vi "AB_820_850_Project_Source_ExportedVI.vi"(6 "dataForPrevious":T2, 7 "action":T6, 8 "error in (no error)":errorcluster, 9 "index in":i32, 10 "dataSource in":cluster{"vipInfo":T1}, 11 "buildObject":T5) -> (0 "error out":errorcluster, 1 "index out":i32, 2 "dataSource out":cluster{"vipInfo":T1}, 3 "buildObject out":T5)   [LabVIEW 2020]
doc: "Reads and writes the data to the object property bag."
uses:
  <resource>/Framework/Providers/API/ItemRef.ctl
  <vilib>/AppBuilder/RW_Project/AB_RW_Project_PropBag_Action.ctl
  <vilib>/AppBuilder/RW_Project/AB_RW_Project_Source_Data_for_Previous.ctl
  <vilib>/AppBuilder/AB_BuildType.ctl
  <vilib>/Utility/lvfile.llb/LVFileType.ctl
  <vilib>/AppBuilder/ABAPI Dist VI Proto Info.ctl
  <vilib>/Utility/lvfile.llb/NI_FileType.lvlib
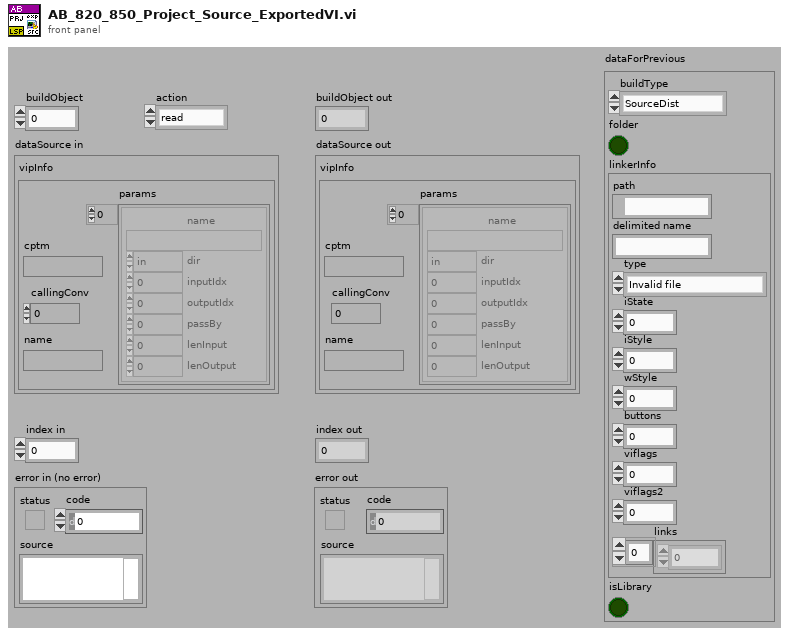
[diagram p1: front panel]
types:
  T1 = typedef "ABAPI Dist VI Proto Info.ctl" = cluster{"cptm":string, "params":cluster{"name":string, "dir":enum32{"in", "out", "in/out", "length"}, "inputIdx":i32, "outputIdx":i32, "passBy":i32, "lenInput":i32, "lenOutput":i32}[], "callingConv":i32, "name":string}
  T2 = typedef "AB_RW_Project_Source_Data_for_Previous.ctl" = cluster{"buildType":T3, "folder":bool, "linkerInfo":cluster{"path":path, "delimited name":string, "type":T4, "iState":u32, "iStyle":u16, "wStyle":u16, "buttons":u16, "viflags":u32, "viflags2":u32, "links":u32[]}, "isLibrary":bool}
  T3 = typedef "AB_BuildType.ctl" = enum16{"SourceDist", "EXE", "DLL", "RTExe"}
  T4 = typedef "NI_FileType.lvlib/LVFileType.ctl" = enum32{"Invalid file", "Unknown type", "Instrument", "Control", "Polymorphic VI", "Project", "Library", "LVClass", "XControl", "XNode", "Shared library", ".NET assembly", "ActiveX interface", "CIN", "Run-time menu", "Palette menu", "Help file", "LLB", "XNode Edit Dependency", "Class Private Data Control", "Statechart", "MathScript .m file", "Ladder Diagram", "LVLibp", "XNode Build Dependency"}
  T5 = typedef "ItemRef.ctl" = u64
  T6 = typedef "AB_RW_Project_PropBag_Action.ctl" = enum16{"read", "write", "clear", "readPrevious", "writePrevious", "clearPrevious"}
  T7 = cluster{"name":string, "dir":enum32{"in", "out", "in/out", "length"}, "inputIdx":i32, "outputIdx":i32, "passBy":i32, "lenInput":i32, "lenOutput":i32}
  T8 = cluster{"name":string, "dir":enum32{"in", "out", "in/out", "length"}, "inputIdx":i32, "outputIdx":i32, "passBy":i32, "lenInput":i32, "lenOutput":i32}[]
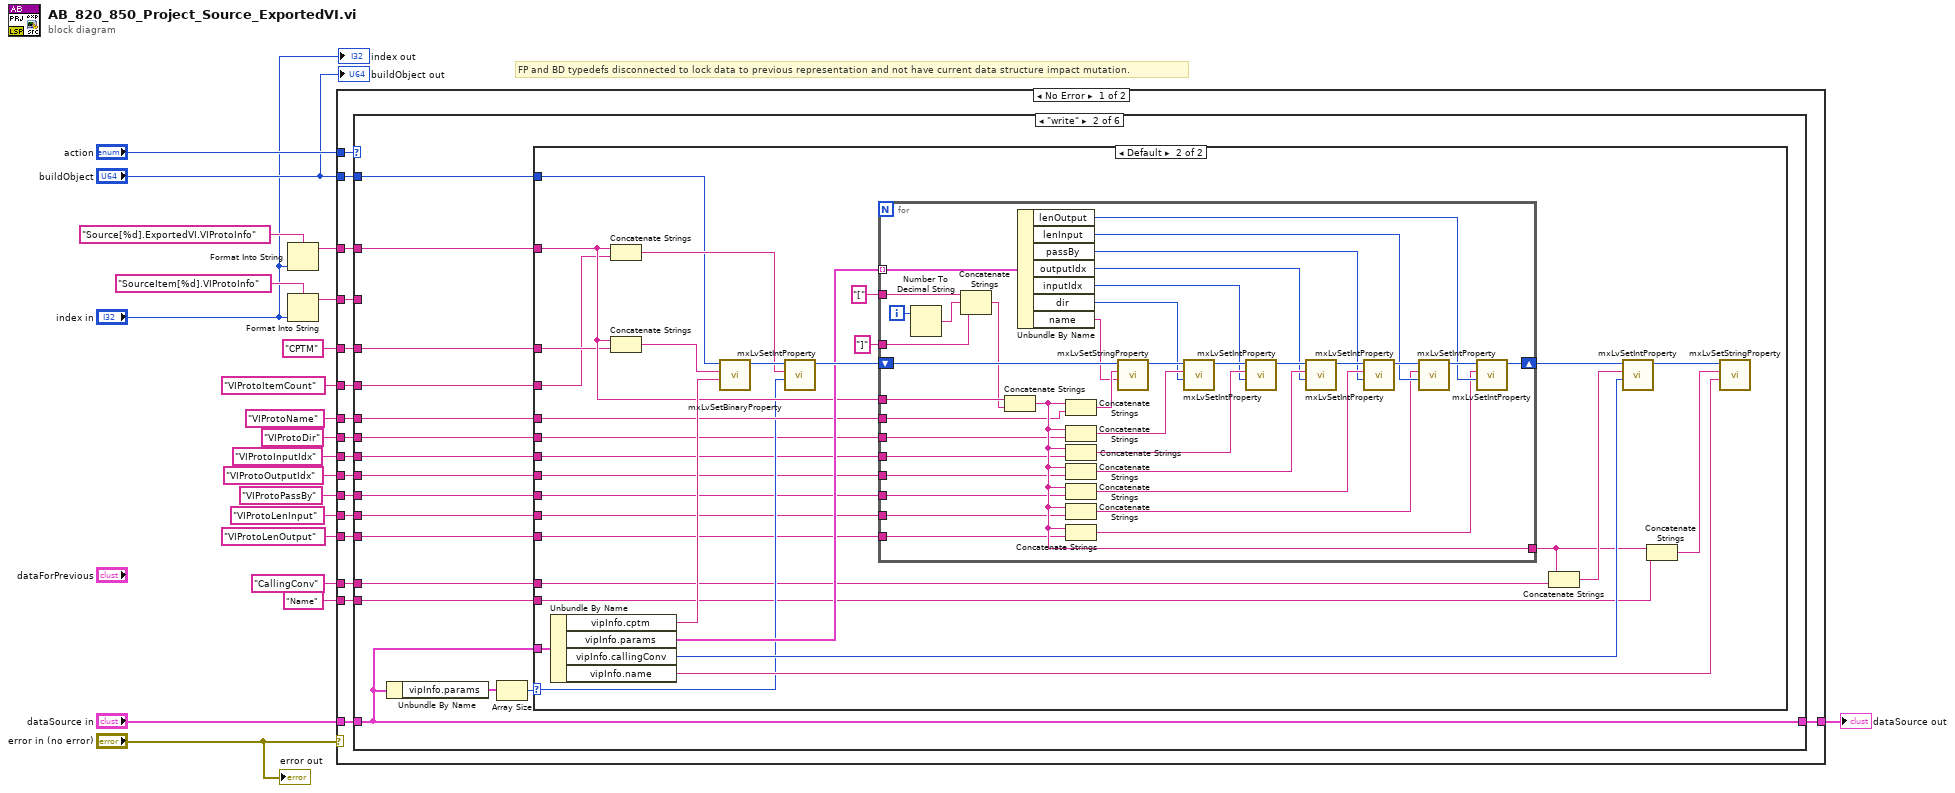
[diagram p0: block diagram]
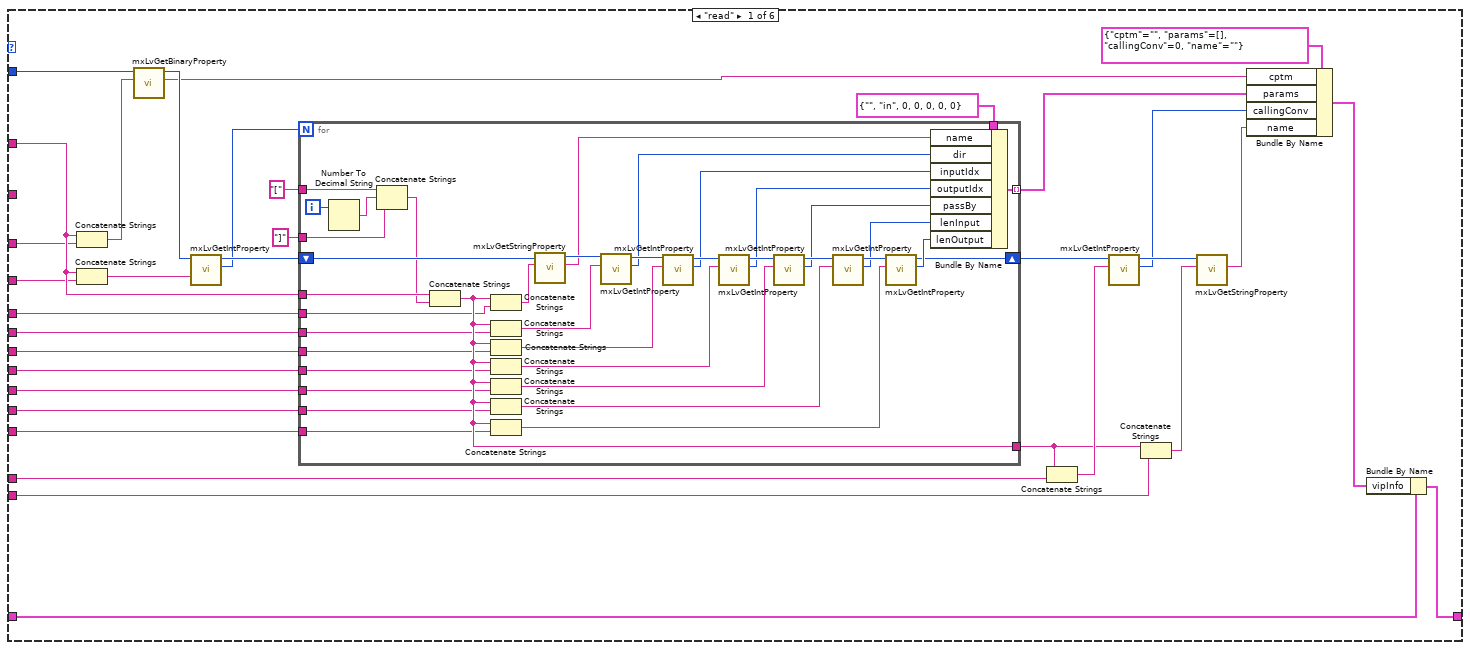
[diagram p2: hidden frame]
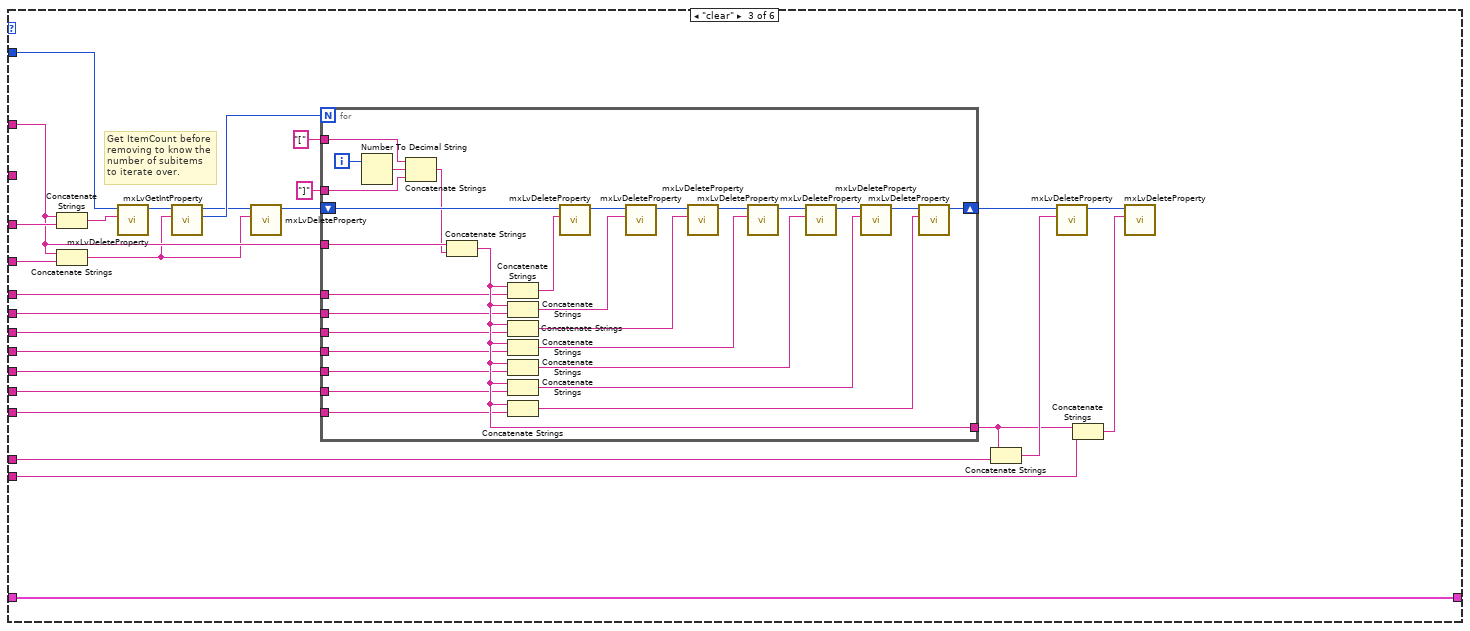
[diagram p4: hidden frame]
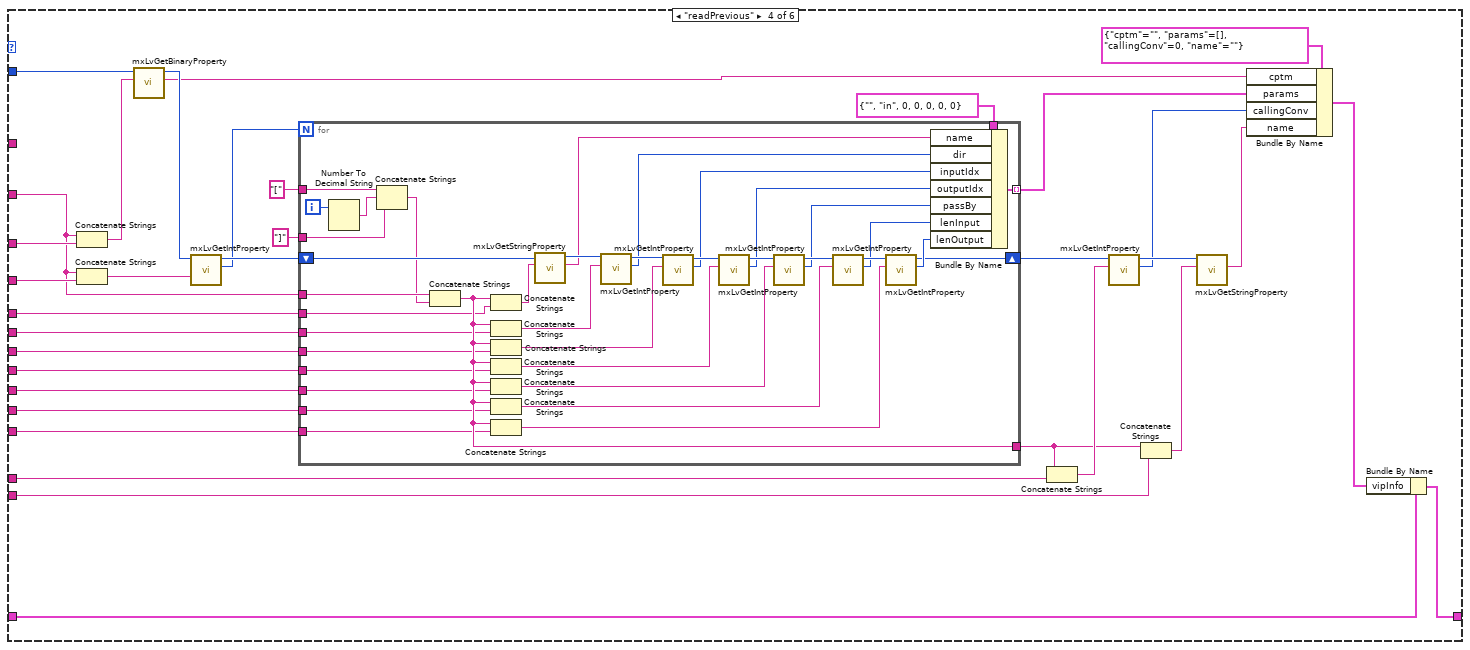
[diagram p5: hidden frame]
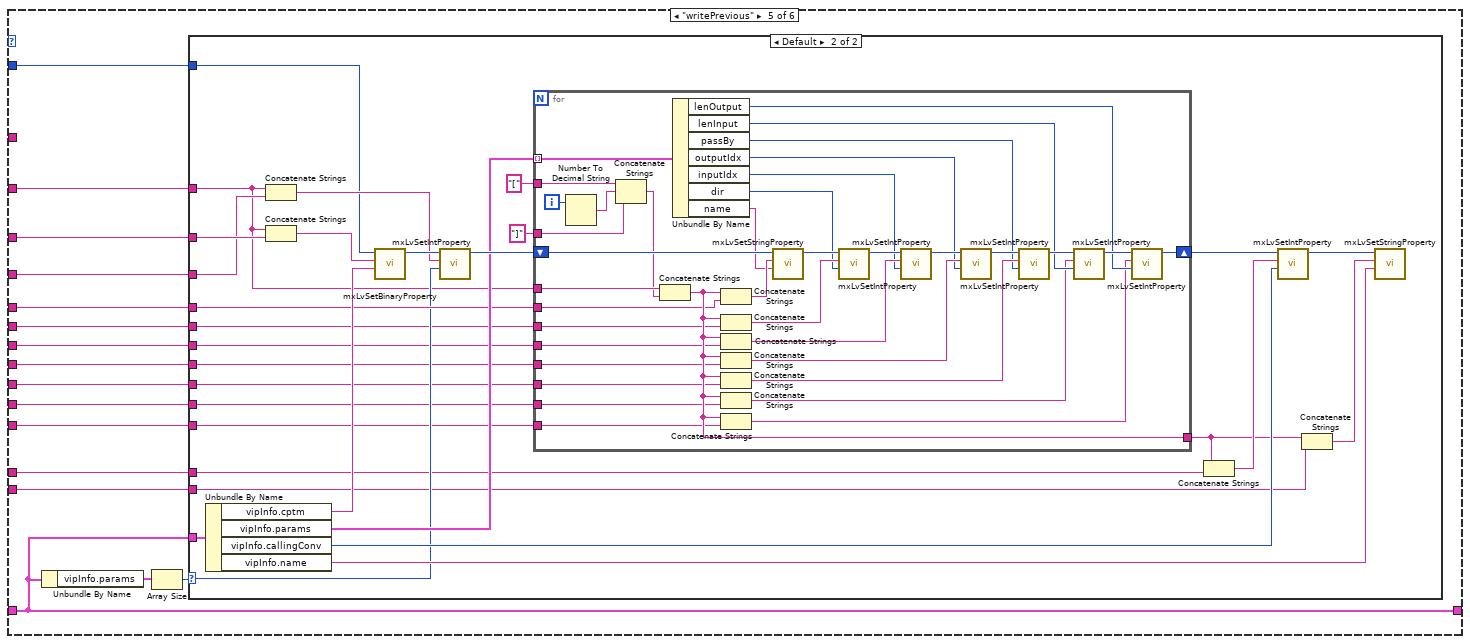
[diagram p6: hidden frame]
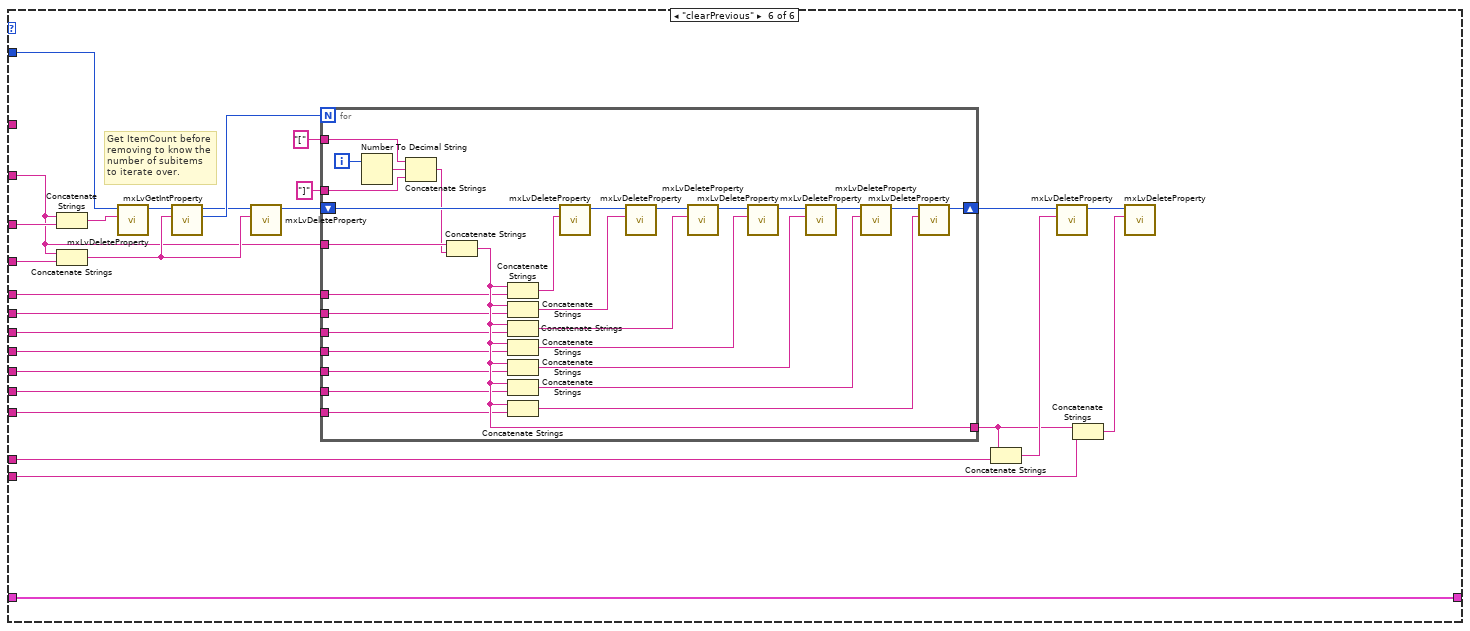
[diagram p8: hidden frame]
diagram:
  # "FP and BD typedefs disconnected to lock data to previous representation and not have current data structure impact mutation."
  n1 = Format Into String(format string="Source[%d].ExportedVI.VIProtoInfo", "index in") -> (resulting string=w19:string)  [unwired: 2 in, 1 out]
  n2 = Format Into String(format string="SourceItem[%d].VIProtoInfo", "index in") -> (resulting string=w17:string)  [unwired: 2 in, 1 out]
  n3 = case shown="No Error" "error in (no error)" {
    tunnel: "action" -> [w38 _]
    tunnel: "dataSource in" -> [w37 w461]
    tunnel: w19 -> [w36 _]
    tunnel: w17 -> [w35 _]
    tunnel: "buildObject" -> [w34 _]
    tunnel: [w33 w461] -> w12
    tunnel: "CPTM" -> [w32 _]
    tunnel: "VIProtoItemCount" -> [w31 _]
    tunnel: "VIProtoName" ("string") -> [w30 _]
    tunnel: "VIProtoDir" ("string") -> [w29 _]
    tunnel: "VIProtoInputIdx" ("string") -> [w28 _]
    tunnel: "VIProtoOutputIdx" ("string") -> [w27 _]
    tunnel: "VIProtoPassBy" ("string") -> [w26 _]
    tunnel: "VIProtoLenInput" ("string") -> [w25 _]
    tunnel: "VIProtoLenOutput" ("string") -> [w24 _]
    tunnel: "CallingConv" -> [w23 _]
    tunnel: "Name" -> [w22 _]
    frame No Error {
      n4 = case shown="\"write\"" w38 {
        tunnel: w34 -> [w69 w124 w217 w281 w336 w429]
        tunnel: w37 -> [w72 w119 w220 w283 w331 w431]
        tunnel: w36 -> [w70 w125 w218 _ _ _]
        tunnel: w35 -> [_ _ _ w250 w322 w405]
        tunnel: [w71 w119 w220 w282 w331 w431] -> w33
        tunnel: w32 -> [w49 w122 w219 w261 w334 w430]
        tunnel: w31 -> [w48 w121 w216 w260 w333 w428]
        tunnel: w30 -> [w47 w123 w202 w259 w335 w414]
        tunnel: w29 -> [w46 w118 w201 w258 w330 w413]
        tunnel: w28 -> [w45 w117 w200 w257 w329 w412]
        tunnel: w27 -> [w44 w116 w199 w256 w328 w411]
        tunnel: w26 -> [w43 w115 w198 w255 w327 w410]
        tunnel: w25 -> [w42 w114 w197 w254 w326 w409]
        tunnel: w24 -> [w41 w113 w196 w253 w325 w408]
        tunnel: w23 -> [w40 w112 w194 w252 w324 w406]
        tunnel: w22 -> [w39 w111 w195 w251 w323 w407]
        frame "read" {
          n5 = Concatenate Strings(w70, w49) -> (w66:string)
          n6 = Concatenate Strings(w70, w48) -> (w62:string)
          n7 = call <resource>:"mxLvGetBinaryProperty.vi"("Tag"=w66, "Item"=w69) -> ("Value"=w50:string, "Item"=w63:T5)  [unwired: 7 in, 1 out]
          n8 = call <resource>:"mxLvGetIntProperty.vi"("Tag"=w62, "Item"=w63) -> ("Value"=w56:i32, "Item"=w61:T5)  [unwired: 7 in, 1 out]
          n9 = for {
            N: w56 -> [_]
            tunnel: "[" -> [w109]
            tunnel: "]" -> [w108]
            tunnel: w70 -> [w103]
            tunnel: [w90] -> w57
            tunnel: T7 {"name"="", "dir"=enum."in", "inputIdx"=0, "outputIdx"=0, "passBy"=0, "lenInput"=0, "lenOutput"=0} -> [w89]
            tunnel: [w81] -> w53 mode=indexing
            shift-right: [w80] -> w51
            shift-left: w61 -> [w106]
            tunnel: w47 -> [w79]
            tunnel: w46 -> [w78]
            tunnel: w45 -> [w77]
            tunnel: w44 -> [w76]
            tunnel: w43 -> [w75]
            tunnel: w42 -> [w74]
            tunnel: w41 -> [w73]
            i -> [w107]
            n10 = Number To Decimal String(number=w107) -> (decimal integer string=w110:string)  [unwired: 1 in]
            n11 = Concatenate Strings(w109, w110, w108) -> (w102:string)
            n12 = Concatenate Strings(w103, w102) -> (w90:string)
            n13 = Concatenate Strings(w90, w79) -> (w105:string)
            n14 = Concatenate Strings(w90, w78) -> (w101:string)
            n15 = Concatenate Strings(w90, w77) -> (w100:string)
            n16 = Concatenate Strings(w90, w76) -> (w94:string)
            n17 = Concatenate Strings(w90, w75) -> (w93:string)
            n18 = Concatenate Strings(w90, w74) -> (w92:string)
            n19 = Concatenate Strings(w90, w73) -> (w91:string)
            n20 = call <resource>:"mxLvGetStringProperty.vi"("Tag"=w105, "Item"=w106) -> ("Value"=w88:string, "Item"=w104:T5)  [unwired: 7 in, 1 out]
            n21 = call <resource>:"mxLvGetIntProperty.vi"("Tag"=w101, "Item"=w104) -> ("Value"=w87:i32, "Item"=w99:T5)  [unwired: 7 in, 1 out]
            n22 = call <resource>:"mxLvGetIntProperty.vi"("Tag"=w100, "Item"=w99) -> ("Value"=w86:i32, "Item"=w98:T5)  [unwired: 7 in, 1 out]
            n23 = call <resource>:"mxLvGetIntProperty.vi"("Tag"=w94, "Item"=w98) -> ("Value"=w85:i32, "Item"=w97:T5)  [unwired: 7 in, 1 out]
            n24 = call <resource>:"mxLvGetIntProperty.vi"("Tag"=w93, "Item"=w97) -> ("Value"=w84:i32, "Item"=w96:T5)  [unwired: 7 in, 1 out]
            n25 = call <resource>:"mxLvGetIntProperty.vi"("Tag"=w92, "Item"=w96) -> ("Value"=w83:i32, "Item"=w95:T5)  [unwired: 7 in, 1 out]
            n26 = call <resource>:"mxLvGetIntProperty.vi"("Tag"=w91, "Item"=w95) -> ("Value"=w82:i32, "Item"=w80:T5)  [unwired: 7 in, 1 out]
            n27 = Bundle By Name(cluster=w89, "name"=w88, "dir"=w87, "inputIdx"=w86, "outputIdx"=w85, "passBy"=w84, "lenInput"=w83, "lenOutput"=w82) -> (w81:T7)
          }
          n28 = Concatenate Strings(w57, w40) -> (w64:string)
          n29 = call <resource>:"mxLvGetIntProperty.vi"("Tag"=w64, "Item"=w51) -> ("Value"=w54:i32, "Item"=w58:T5)  [unwired: 7 in, 1 out]
          n30 = Concatenate Strings(w57, w39) -> (w65:string)
          n31 = call <resource>:"mxLvGetStringProperty.vi"("Tag"=w65, "Item"=w58) -> ("Value"=w52:string)  [unwired: 7 in, 2 out]
          n32 = Bundle By Name(cluster=T1 {"cptm"="", "params"=[], "callingConv"=0, "name"=""} ("vipInfo"), "cptm"=w50, "params"=w53, "callingConv"=w54, "name"=w52) -> (w67:T1)
          n33 = Bundle By Name(cluster=w72, "vipInfo"=w67) -> (w71:cluster{"vipInfo":T1})
        }
        frame "write" {
          n34 = Unbundle By Name(w119) -> ("vipInfo.params"=w126:T8)
          n35 = Array Size(array=w126) -> (size(s)=w120:i32)
          n36 = case shown="Default" w120 {
            selector: w120 -> [_ w135]
            tunnel: w124 -> [_ w141]
            tunnel: w119 -> [_ w140]
            tunnel: w125 -> [_ w139]
            tunnel: w123 -> [_ w138]
            tunnel: w122 -> [_ w137]
            tunnel: w121 -> [_ w136]
            tunnel: w118 -> [_ w134]
            tunnel: w117 -> [_ w133]
            tunnel: w116 -> [_ w132]
            tunnel: w115 -> [_ w131]
            tunnel: w114 -> [_ w130]
            tunnel: w113 -> [_ w129]
            tunnel: w112 -> [_ w128]
            tunnel: w111 -> [_ w127]
            frame 0 {
              # "If default, then don't write anything out."
            }
            frame Default {
              n37 = Unbundle By Name(w140) -> ("vipInfo.cptm"=w155:string, "vipInfo.params"=w147:T8, "vipInfo.callingConv"=w151:i32, "vipInfo.name"=w152:string)
              n38 = Concatenate Strings(w139, w136) -> (w149:string)
              n39 = Concatenate Strings(w139, w137) -> (w156:string)
              n40 = call <resource>:"mxLvSetBinaryProperty.vi"("Value"=w155, "Tag"=w156, "Item"=w141) -> ("Item"=w150:T5)  [unwired: 7 in, 1 out]
              n41 = call <resource>:"mxLvSetIntProperty.vi"("Value (0)"=w135, "Tag"=w149, "Item"=w150) -> ("Item"=w148:T5)  [unwired: 7 in, 1 out]
              n42 = for {
                tunnel: w147 -> [w193] mode=indexing
                tunnel: "[" -> [w191]
                tunnel: "]" -> [w190]
                tunnel: w139 -> [w184]
                tunnel: [w165] -> w142
                shift-right: [w164] -> w144
                shift-left: w148 -> [w188]
                tunnel: w138 -> [w163]
                tunnel: w134 -> [w162]
                tunnel: w133 -> [w161]
                tunnel: w132 -> [w160]
                tunnel: w131 -> [w159]
                tunnel: w130 -> [w158]
                tunnel: w129 -> [w157]
                i -> [w189]
                n43 = Number To Decimal String(number=w189) -> (decimal integer string=w192:string)  [unwired: 1 in]
                n44 = Concatenate Strings(w191, w192, w190) -> (w183:string)
                n45 = Concatenate Strings(w184, w183) -> (w165:string)
                n46 = Unbundle By Name(w193) -> ("lenOutput"=w167:i32, "lenInput"=w169:i32, "passBy"=w170:i32, "outputIdx"=w171:i32, "inputIdx"=w178:i32, "dir"=w181:enum32{"in", "out", "in/out", "length"}, "name"=w186:string)
                n47 = Concatenate Strings(w165, w163) -> (w187:string)
                n48 = Concatenate Strings(w165, w162) -> (w182:string)
                n49 = Concatenate Strings(w165, w161) -> (w180:string)
                n50 = Concatenate Strings(w165, w160) -> (w173:string)
                n51 = Concatenate Strings(w165, w159) -> (w172:string)
                n52 = Concatenate Strings(w165, w158) -> (w168:string)
                n53 = Concatenate Strings(w165, w157) -> (w166:string)
                n54 = call <resource>:"mxLvSetStringProperty.vi"("Value (\"\")"=w186, "Tag"=w187, "Item"=w188) -> ("Item"=w185:T5)  [unwired: 7 in, 1 out]
                n55 = call <resource>:"mxLvSetIntProperty.vi"("Value (0)"=w181, "Tag"=w182, "Item"=w185) -> ("Item"=w179:T5)  [unwired: 7 in, 1 out]
                n56 = call <resource>:"mxLvSetIntProperty.vi"("Value (0)"=w178, "Tag"=w180, "Item"=w179) -> ("Item"=w177:T5)  [unwired: 7 in, 1 out]
                n57 = call <resource>:"mxLvSetIntProperty.vi"("Value (0)"=w171, "Tag"=w173, "Item"=w177) -> ("Item"=w176:T5)  [unwired: 7 in, 1 out]
                n58 = call <resource>:"mxLvSetIntProperty.vi"("Value (0)"=w170, "Tag"=w172, "Item"=w176) -> ("Item"=w175:T5)  [unwired: 7 in, 1 out]
                n59 = call <resource>:"mxLvSetIntProperty.vi"("Value (0)"=w169, "Tag"=w168, "Item"=w175) -> ("Item"=w174:T5)  [unwired: 7 in, 1 out]
                n60 = call <resource>:"mxLvSetIntProperty.vi"("Value (0)"=w167, "Tag"=w166, "Item"=w174) -> ("Item"=w164:T5)  [unwired: 7 in, 1 out]
              }
              n61 = Concatenate Strings(w142, w128) -> (w153:string)
              n62 = call <resource>:"mxLvSetIntProperty.vi"("Value (0)"=w151, "Tag"=w153, "Item"=w144) -> ("Item"=w143:T5)  [unwired: 7 in, 1 out]
              n63 = Concatenate Strings(w142, w127) -> (w154:string)
              n64 = call <resource>:"mxLvSetStringProperty.vi"("Value (\"\")"=w152, "Tag"=w154, "Item"=w143) -> ()  [unwired: 7 in, 2 out]
            }
          }
        }
        frame "clear" {
          # "Get ItemCount before removing to know the number of subitems to iterate over."
          n65 = Concatenate Strings(w218, w219) -> (w215:string)
          n66 = Concatenate Strings(w218, w216) -> (w203:string)
          n67 = call <resource>:"mxLvDeleteProperty.vi"("Tag"=w215, "Item"=w217) -> ("Item"=w205:T5)  [unwired: 8 in, 1 out]
          n68 = call <resource>:"mxLvGetIntProperty.vi"("Tag"=w203, "Item"=w205) -> ("Value"=w206:i32, "Item"=w204:T5)  [unwired: 7 in, 1 out]
          n69 = call <resource>:"mxLvDeleteProperty.vi"("Tag"=w203, "Item"=w204) -> ("Item"=w212:T5)  [unwired: 8 in, 1 out]
          n70 = for {
            N: w206 -> [_]
            tunnel: "[" -> [w248]
            tunnel: "]" -> [w247]
            tunnel: w218 -> [w242]
            tunnel: [w229] -> w207
            shift-right: [w228] -> w209
            shift-left: w212 -> [w245]
            tunnel: w202 -> [w227]
            tunnel: w201 -> [w226]
            tunnel: w200 -> [w225]
            tunnel: w199 -> [w224]
            tunnel: w198 -> [w223]
            tunnel: w197 -> [w222]
            tunnel: w196 -> [w221]
            i -> [w246]
            n71 = Number To Decimal String(number=w246) -> (decimal integer string=w249:string)  [unwired: 1 in]
            n72 = Concatenate Strings(w248, w249, w247) -> (w241:string)
            n73 = Concatenate Strings(w242, w241) -> (w229:string)
            n74 = Concatenate Strings(w229, w227) -> (w244:string)
            n75 = Concatenate Strings(w229, w226) -> (w240:string)
            n76 = Concatenate Strings(w229, w225) -> (w239:string)
            n77 = Concatenate Strings(w229, w224) -> (w233:string)
            n78 = Concatenate Strings(w229, w223) -> (w232:string)
            n79 = Concatenate Strings(w229, w222) -> (w231:string)
            n80 = Concatenate Strings(w229, w221) -> (w230:string)
            n81 = call <resource>:"mxLvDeleteProperty.vi"("Tag"=w244, "Item"=w245) -> ("Item"=w243:T5)  [unwired: 8 in, 1 out]
            n82 = call <resource>:"mxLvDeleteProperty.vi"("Tag"=w240, "Item"=w243) -> ("Item"=w238:T5)  [unwired: 8 in, 1 out]
            n83 = call <resource>:"mxLvDeleteProperty.vi"("Tag"=w239, "Item"=w238) -> ("Item"=w237:T5)  [unwired: 8 in, 1 out]
            n84 = call <resource>:"mxLvDeleteProperty.vi"("Tag"=w233, "Item"=w237) -> ("Item"=w236:T5)  [unwired: 8 in, 1 out]
            n85 = call <resource>:"mxLvDeleteProperty.vi"("Tag"=w232, "Item"=w236) -> ("Item"=w235:T5)  [unwired: 8 in, 1 out]
            n86 = call <resource>:"mxLvDeleteProperty.vi"("Tag"=w231, "Item"=w235) -> ("Item"=w234:T5)  [unwired: 8 in, 1 out]
            n87 = call <resource>:"mxLvDeleteProperty.vi"("Tag"=w230, "Item"=w234) -> ("Item"=w228:T5)  [unwired: 8 in, 1 out]
          }
          n88 = Concatenate Strings(w207, w194) -> (w213:string)
          n89 = call <resource>:"mxLvDeleteProperty.vi"("Tag"=w213, "Item"=w209) -> ("Item"=w208:T5)  [unwired: 8 in, 1 out]
          n90 = Concatenate Strings(w207, w195) -> (w214:string)
          n91 = call <resource>:"mxLvDeleteProperty.vi"("Tag"=w214, "Item"=w208) -> ()  [unwired: 8 in, 2 out]
        }
        frame "readPrevious" {
          n92 = Concatenate Strings(w250, w261) -> (w278:string)
          n93 = Concatenate Strings(w250, w260) -> (w274:string)
          n94 = call <resource>:"mxLvGetBinaryProperty.vi"("Tag"=w278, "Item"=w281) -> ("Value"=w262:string, "Item"=w275:T5)  [unwired: 7 in, 1 out]
          n95 = call <resource>:"mxLvGetIntProperty.vi"("Tag"=w274, "Item"=w275) -> ("Value"=w268:i32, "Item"=w273:T5)  [unwired: 7 in, 1 out]
          n96 = for {
            N: w268 -> [_]
            tunnel: "[" -> [w320]
            tunnel: "]" -> [w319]
            tunnel: w250 -> [w314]
            tunnel: [w301] -> w269
            tunnel: T7 {"name"="", "dir"=enum."in", "inputIdx"=0, "outputIdx"=0, "passBy"=0, "lenInput"=0, "lenOutput"=0} -> [w300]
            tunnel: [w292] -> w265 mode=indexing
            shift-right: [w291] -> w263
            shift-left: w273 -> [w317]
            tunnel: w259 -> [w290]
            tunnel: w258 -> [w289]
            tunnel: w257 -> [w288]
            tunnel: w256 -> [w287]
            tunnel: w255 -> [w286]
            tunnel: w254 -> [w285]
            tunnel: w253 -> [w284]
            i -> [w318]
            n97 = Number To Decimal String(number=w318) -> (decimal integer string=w321:string)  [unwired: 1 in]
            n98 = Concatenate Strings(w320, w321, w319) -> (w313:string)
            n99 = Concatenate Strings(w314, w313) -> (w301:string)
            n100 = Concatenate Strings(w301, w290) -> (w316:string)
            n101 = Concatenate Strings(w301, w289) -> (w312:string)
            n102 = Concatenate Strings(w301, w288) -> (w311:string)
            n103 = Concatenate Strings(w301, w287) -> (w305:string)
            n104 = Concatenate Strings(w301, w286) -> (w304:string)
            n105 = Concatenate Strings(w301, w285) -> (w303:string)
            n106 = Concatenate Strings(w301, w284) -> (w302:string)
            n107 = call <resource>:"mxLvGetStringProperty.vi"("Tag"=w316, "Item"=w317) -> ("Value"=w299:string, "Item"=w315:T5)  [unwired: 7 in, 1 out]
            n108 = call <resource>:"mxLvGetIntProperty.vi"("Tag"=w312, "Item"=w315) -> ("Value"=w298:i32, "Item"=w310:T5)  [unwired: 7 in, 1 out]
            n109 = call <resource>:"mxLvGetIntProperty.vi"("Tag"=w311, "Item"=w310) -> ("Value"=w297:i32, "Item"=w309:T5)  [unwired: 7 in, 1 out]
            n110 = call <resource>:"mxLvGetIntProperty.vi"("Tag"=w305, "Item"=w309) -> ("Value"=w296:i32, "Item"=w308:T5)  [unwired: 7 in, 1 out]
            n111 = call <resource>:"mxLvGetIntProperty.vi"("Tag"=w304, "Item"=w308) -> ("Value"=w295:i32, "Item"=w307:T5)  [unwired: 7 in, 1 out]
            n112 = call <resource>:"mxLvGetIntProperty.vi"("Tag"=w303, "Item"=w307) -> ("Value"=w294:i32, "Item"=w306:T5)  [unwired: 7 in, 1 out]
            n113 = call <resource>:"mxLvGetIntProperty.vi"("Tag"=w302, "Item"=w306) -> ("Value"=w293:i32, "Item"=w291:T5)  [unwired: 7 in, 1 out]
            n114 = Bundle By Name(cluster=w300, "name"=w299, "dir"=w298, "inputIdx"=w297, "outputIdx"=w296, "passBy"=w295, "lenInput"=w294, "lenOutput"=w293) -> (w292:T7)
          }
          n115 = Concatenate Strings(w269, w252) -> (w276:string)
          n116 = call <resource>:"mxLvGetIntProperty.vi"("Tag"=w276, "Item"=w263) -> ("Value"=w266:i32, "Item"=w270:T5)  [unwired: 7 in, 1 out]
          n117 = Concatenate Strings(w269, w251) -> (w277:string)
          n118 = call <resource>:"mxLvGetStringProperty.vi"("Tag"=w277, "Item"=w270) -> ("Value"=w264:string)  [unwired: 7 in, 2 out]
          n119 = Bundle By Name(cluster=T1 {"cptm"="", "params"=[], "callingConv"=0, "name"=""} ("vipInfo"), "cptm"=w262, "params"=w265, "callingConv"=w266, "name"=w264) -> (w279:T1)
          n120 = Bundle By Name(cluster=w283, "vipInfo"=w279) -> (w282:cluster{"vipInfo":T1})
        }
        frame "writePrevious" {
          n121 = Unbundle By Name(w331) -> ("vipInfo.params"=w337:T8)
          n122 = Array Size(array=w337) -> (size(s)=w332:i32)
          n123 = case shown="Default" w332 {
            selector: w332 -> [_ w347]
            tunnel: w336 -> [_ w352]
            tunnel: w331 -> [_ w351]
            tunnel: w335 -> [_ w350]
            tunnel: w334 -> [_ w349]
            tunnel: w333 -> [_ w348]
            tunnel: w330 -> [_ w346]
            tunnel: w329 -> [_ w345]
            tunnel: w328 -> [_ w344]
            tunnel: w327 -> [_ w343]
            tunnel: w326 -> [_ w342]
            tunnel: w325 -> [_ w341]
            tunnel: w324 -> [_ w340]
            tunnel: w323 -> [_ w339]
            tunnel: w322 -> [_ w338]
            frame 0 {
              # "If default, then don't write anything out."
            }
            frame Default {
              n124 = Unbundle By Name(w351) -> ("vipInfo.cptm"=w366:string, "vipInfo.params"=w358:T8, "vipInfo.callingConv"=w362:i32, "vipInfo.name"=w363:string)
              n125 = Concatenate Strings(w338, w348) -> (w360:string)
              n126 = Concatenate Strings(w338, w349) -> (w367:string)
              n127 = call <resource>:"mxLvSetBinaryProperty.vi"("Value"=w366, "Tag"=w367, "Item"=w352) -> ("Item"=w361:T5)  [unwired: 7 in, 1 out]
              n128 = call <resource>:"mxLvSetIntProperty.vi"("Value (0)"=w347, "Tag"=w360, "Item"=w361) -> ("Item"=w359:T5)  [unwired: 7 in, 1 out]
              n129 = for {
                tunnel: w358 -> [w404] mode=indexing
                tunnel: "[" -> [w402]
                tunnel: "]" -> [w401]
                tunnel: w338 -> [w395]
                tunnel: [w376] -> w353
                shift-right: [w375] -> w355
                shift-left: w359 -> [w399]
                tunnel: w350 -> [w374]
                tunnel: w346 -> [w373]
                tunnel: w345 -> [w372]
                tunnel: w344 -> [w371]
                tunnel: w343 -> [w370]
                tunnel: w342 -> [w369]
                tunnel: w341 -> [w368]
                i -> [w400]
                n130 = Number To Decimal String(number=w400) -> (decimal integer string=w403:string)  [unwired: 1 in]
                n131 = Concatenate Strings(w402, w403, w401) -> (w394:string)
                n132 = Concatenate Strings(w395, w394) -> (w376:string)
                n133 = Unbundle By Name(w404) -> ("lenOutput"=w378:i32, "lenInput"=w380:i32, "passBy"=w381:i32, "outputIdx"=w382:i32, "inputIdx"=w389:i32, "dir"=w392:enum32{"in", "out", "in/out", "length"}, "name"=w397:string)
                n134 = Concatenate Strings(w376, w374) -> (w398:string)
                n135 = Concatenate Strings(w376, w373) -> (w393:string)
                n136 = Concatenate Strings(w376, w372) -> (w391:string)
                n137 = Concatenate Strings(w376, w371) -> (w384:string)
                n138 = Concatenate Strings(w376, w370) -> (w383:string)
                n139 = Concatenate Strings(w376, w369) -> (w379:string)
                n140 = Concatenate Strings(w376, w368) -> (w377:string)
                n141 = call <resource>:"mxLvSetStringProperty.vi"("Value (\"\")"=w397, "Tag"=w398, "Item"=w399) -> ("Item"=w396:T5)  [unwired: 7 in, 1 out]
                n142 = call <resource>:"mxLvSetIntProperty.vi"("Value (0)"=w392, "Tag"=w393, "Item"=w396) -> ("Item"=w390:T5)  [unwired: 7 in, 1 out]
                n143 = call <resource>:"mxLvSetIntProperty.vi"("Value (0)"=w389, "Tag"=w391, "Item"=w390) -> ("Item"=w388:T5)  [unwired: 7 in, 1 out]
                n144 = call <resource>:"mxLvSetIntProperty.vi"("Value (0)"=w382, "Tag"=w384, "Item"=w388) -> ("Item"=w387:T5)  [unwired: 7 in, 1 out]
                n145 = call <resource>:"mxLvSetIntProperty.vi"("Value (0)"=w381, "Tag"=w383, "Item"=w387) -> ("Item"=w386:T5)  [unwired: 7 in, 1 out]
                n146 = call <resource>:"mxLvSetIntProperty.vi"("Value (0)"=w380, "Tag"=w379, "Item"=w386) -> ("Item"=w385:T5)  [unwired: 7 in, 1 out]
                n147 = call <resource>:"mxLvSetIntProperty.vi"("Value (0)"=w378, "Tag"=w377, "Item"=w385) -> ("Item"=w375:T5)  [unwired: 7 in, 1 out]
              }
              n148 = Concatenate Strings(w353, w340) -> (w364:string)
              n149 = call <resource>:"mxLvSetIntProperty.vi"("Value (0)"=w362, "Tag"=w364, "Item"=w355) -> ("Item"=w354:T5)  [unwired: 7 in, 1 out]
              n150 = Concatenate Strings(w353, w339) -> (w365:string)
              n151 = call <resource>:"mxLvSetStringProperty.vi"("Value (\"\")"=w363, "Tag"=w365, "Item"=w354) -> ()  [unwired: 7 in, 2 out]
            }
          }
        }
        frame "clearPrevious" {
          # "Get ItemCount before removing to know the number of subitems to iterate over."
          n152 = Concatenate Strings(w405, w430) -> (w427:string)
          n153 = Concatenate Strings(w405, w428) -> (w415:string)
          n154 = call <resource>:"mxLvDeleteProperty.vi"("Tag"=w427, "Item"=w429) -> ("Item"=w417:T5)  [unwired: 8 in, 1 out]
          n155 = call <resource>:"mxLvGetIntProperty.vi"("Tag"=w415, "Item"=w417) -> ("Value"=w418:i32, "Item"=w416:T5)  [unwired: 7 in, 1 out]
          n156 = call <resource>:"mxLvDeleteProperty.vi"("Tag"=w415, "Item"=w416) -> ("Item"=w424:T5)  [unwired: 8 in, 1 out]
          n157 = for {
            N: w418 -> [_]
            tunnel: "[" -> [w459]
            tunnel: "]" -> [w458]
            tunnel: w405 -> [w453]
            tunnel: [w440] -> w419
            shift-right: [w439] -> w421
            shift-left: w424 -> [w456]
            tunnel: w414 -> [w438]
            tunnel: w413 -> [w437]
            tunnel: w412 -> [w436]
            tunnel: w411 -> [w435]
            tunnel: w410 -> [w434]
            tunnel: w409 -> [w433]
            tunnel: w408 -> [w432]
            i -> [w457]
            n158 = Number To Decimal String(number=w457) -> (decimal integer string=w460:string)  [unwired: 1 in]
            n159 = Concatenate Strings(w459, w460, w458) -> (w452:string)
            n160 = Concatenate Strings(w453, w452) -> (w440:string)
            n161 = Concatenate Strings(w440, w438) -> (w455:string)
            n162 = Concatenate Strings(w440, w437) -> (w451:string)
            n163 = Concatenate Strings(w440, w436) -> (w450:string)
            n164 = Concatenate Strings(w440, w435) -> (w444:string)
            n165 = Concatenate Strings(w440, w434) -> (w443:string)
            n166 = Concatenate Strings(w440, w433) -> (w442:string)
            n167 = Concatenate Strings(w440, w432) -> (w441:string)
            n168 = call <resource>:"mxLvDeleteProperty.vi"("Tag"=w455, "Item"=w456) -> ("Item"=w454:T5)  [unwired: 8 in, 1 out]
            n169 = call <resource>:"mxLvDeleteProperty.vi"("Tag"=w451, "Item"=w454) -> ("Item"=w449:T5)  [unwired: 8 in, 1 out]
            n170 = call <resource>:"mxLvDeleteProperty.vi"("Tag"=w450, "Item"=w449) -> ("Item"=w448:T5)  [unwired: 8 in, 1 out]
            n171 = call <resource>:"mxLvDeleteProperty.vi"("Tag"=w444, "Item"=w448) -> ("Item"=w447:T5)  [unwired: 8 in, 1 out]
            n172 = call <resource>:"mxLvDeleteProperty.vi"("Tag"=w443, "Item"=w447) -> ("Item"=w446:T5)  [unwired: 8 in, 1 out]
            n173 = call <resource>:"mxLvDeleteProperty.vi"("Tag"=w442, "Item"=w446) -> ("Item"=w445:T5)  [unwired: 8 in, 1 out]
            n174 = call <resource>:"mxLvDeleteProperty.vi"("Tag"=w441, "Item"=w445) -> ("Item"=w439:T5)  [unwired: 8 in, 1 out]
          }
          n175 = Concatenate Strings(w419, w406) -> (w425:string)
          n176 = call <resource>:"mxLvDeleteProperty.vi"("Tag"=w425, "Item"=w421) -> ("Item"=w420:T5)  [unwired: 8 in, 1 out]
          n177 = Concatenate Strings(w419, w407) -> (w426:string)
          n178 = call <resource>:"mxLvDeleteProperty.vi"("Tag"=w426, "Item"=w420) -> ()  [unwired: 8 in, 2 out]
        }
      }
    }
    frame Error {
    }
  }
  "dataSource out" <- w12
  "error out" <- "error in (no error)"
  "buildObject out" <- "buildObject"
  "index out" <- "index in"
